vi "time_name.vi"() -> (0 "time.time()":dbl, 3 "time_format":string)   [LabVIEW 2017]
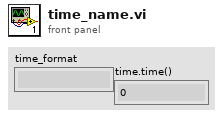
[diagram p1: front panel]
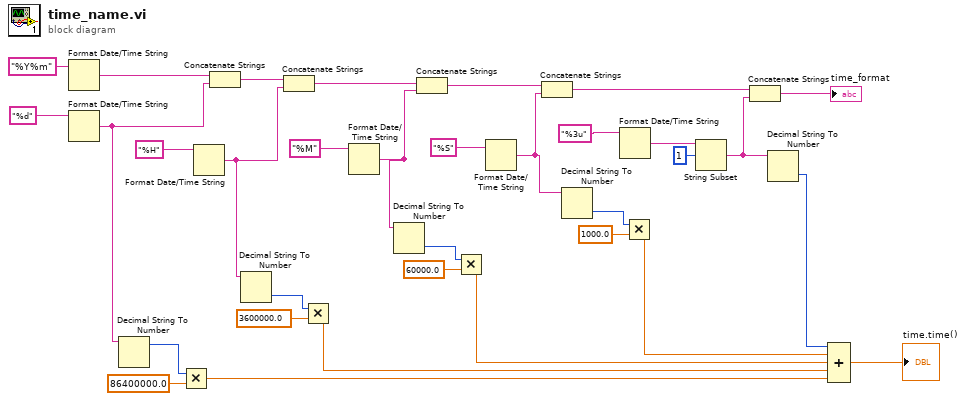
[diagram p0: block diagram]
diagram:
  n1 = Format Date/Time String(time format string (%c)="%Y%m") -> (date/time string=w27:string)  [unwired: 2 in]
  n2 = Format Date/Time String(time format string (%c)="%d") -> (date/time string=w26:string)  [unwired: 2 in]
  n3 = Decimal String To Number(string=w26) -> (offset past number=w24:i32)  [unwired: 2 in, 1 out]
  n4 = Multiply(x=w24, y=86400000.0) -> (x*y=w9:dbl)
  n5 = Format Date/Time String(time format string (%c)="%H") -> (date/time string=w20:string)  [unwired: 2 in]
  n6 = Concatenate Strings(w27, w26) -> (w23:string)
  n7 = Decimal String To Number(string=w20) -> (number=w21:i32)  [unwired: 2 in, 1 out]
  n8 = Concatenate Strings(w23, w20) -> (w19:string)
  n9 = Multiply(x=w21, y=3600000.0) -> (x*y=w8:dbl)
  n10 = Format Date/Time String(time format string (%c)="%M") -> (date/time string=w16:string)  [unwired: 2 in]
  n11 = Decimal String To Number(string=w16) -> (number=w18:i32)  [unwired: 2 in, 1 out]
  n12 = Concatenate Strings(w19, w16) -> (w15:string)
  n13 = Multiply(x=w18, y=60000.0) -> (x*y=w7:dbl)
  n14 = Format Date/Time String(time format string (%c)="%S") -> (date/time string=w12:string)  [unwired: 2 in]
  n15 = Concatenate Strings(w15, w12) -> (w11:string)
  n16 = Decimal String To Number(string=w12) -> (number=w13:i32)  [unwired: 2 in, 1 out]
  n17 = Format Date/Time String(time format string (%c)="%3u") -> (date/time string=w2:string)  [unwired: 2 in]
  n18 = Multiply(x=w13, y=1000.0) -> (x*y=w6:dbl)
  n19 = String Subset(string=w2, offset (0)=1) -> (substring=w1:string)  [unwired: 1 in]
  n20 = Concatenate Strings(w11, w1) -> (→"time_format":string)
  n21 = Decimal String To Number(string=w1) -> (number=w5:i32)  [unwired: 2 in, 1 out]
  n22 = Compound Arithmetic op=ADD(w5, w6, w7, w8, w9) -> (→"time.time()":dbl)
